vi "GOOP_Library_Item_OnPopUpMenu.vi"(11 "Object":u64) -> ()   [LabVIEW 2020]
uses:
  <resource>/Framework/Providers/API/mxLvMenuItem.ctl
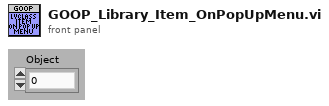
[diagram p1: front panel]
types:
  T1 = typedef "mxLvMenuItem.ctl" = cluster{"Menu Name":string, "Description":string, "Icon File Name":path, "Menu Tag":string, "Enabled":bool, "Checked":bool, "Separator":bool, "Batchable":bool, "Weight":i32, "Batch Mode (Ignored if Not Batchable)":enum32{"Show If All Items Support Command", "Show If Any Items Support Command"}, "Menu Location":enum32{"<None>", "Project", "Project / Build Specifications", "Tools", "Tools / Source Control", "Tools / Real-Time Module", "Help"}, "Exclude From Getting Started Window Menu":bool}
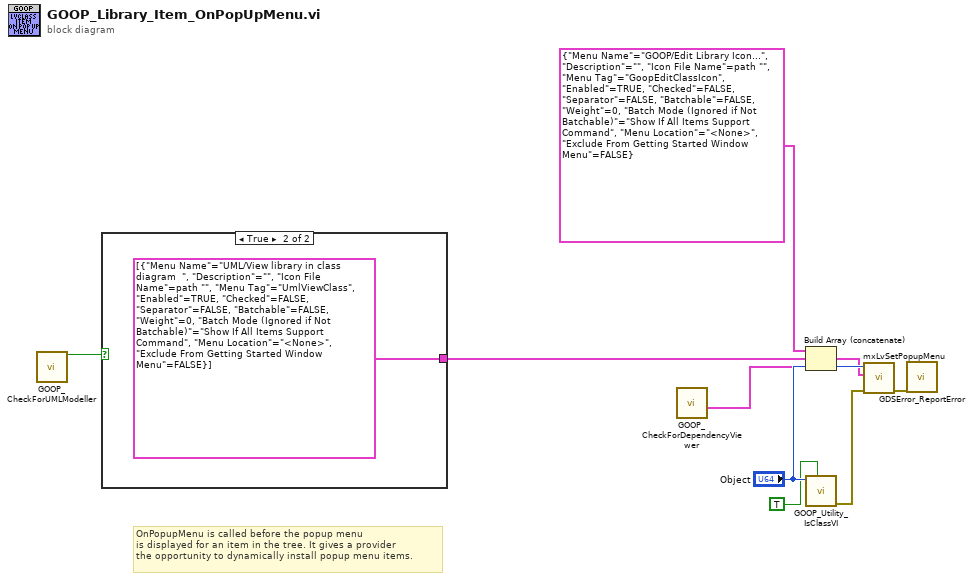
[diagram p0: block diagram]
diagram:
  # "OnPopupMenu is called before the popup menu\nis displayed for an item in the tree. It gives a provider\nthe opportunity to dynamically install popup menu items."
  n1 = call <resource>:"GOOP_CheckForUMLModeller.vi"() -> ("UML Modeller Exists"=w2:bool)  [unwired: 10 in, 1 out]
  n2 = case shown="True" w2 {
    tunnel: [_ T1[] [{"Menu Name"="UML/View library in class diagram  ", "Description"="", "Icon File Name"=path "", "Menu Tag"="UmlViewClass", "Enabled"=TRUE, "Checked"=FALSE, "Separator"=FALSE, "Batchable"=FALSE, "Weight"=0, "Batch Mode (Ignored if Not Batchable)"=enum."Show If All Items Support Command", "Menu Location"=enum."<None>", "Exclude From Getting Started Window Menu"=FALSE}]] -> w6
    frame False {
    }
    frame True {
    }
  }
  n3 = call <resource>:"GOOP_CheckForDependencyViewer.vi"() -> ("PopUpMenu(IfExists)"=w1:T1[])  [unwired: 9 in, 2 out]
  n4 = Build Array (concatenate)(T1 {"Menu Name"="GOOP/Edit Library Icon...", "Description"="", "Icon File Name"=path "", "Menu Tag"="GoopEditClassIcon", "Enabled"=TRUE, "Checked"=FALSE, "Separator"=FALSE, "Batchable"=FALSE, "Weight"=0, "Batch Mode (Ignored if Not Batchable)"=enum."Show If All Items Support Command", "Menu Location"=enum."<None>", "Exclude From Getting Started Window Menu"=FALSE} ("Menu Item"), w6, w1) -> (w7:T1[])
  n5 = call <resource>:"GOOP_Utility_IsClassVI.vi"("KeepClassOpen(False)"=TRUE, "Object"="Object") -> ("error out"=w4:errorcluster)  [unwired: 4 in, 5 out]
  n6 = call <resource>:"mxLvSetPopupMenu.vi"("error in"=w4, "Popup Menu Items"=w7, "Item"="Object") -> ("error out"=w5:errorcluster)  [unwired: 7 in, 1 out]
  n7 = call <resource>:"GDSError_ReportError.vi"("error in (no error)"=w5) -> ()  [unwired: 18 in, 1 out]
